vi "scan_save.vi"(6 "Application ref in":refnum<vi>, 7 "Direction: up/down (T=up)":bool, 8 "error in (no error)":errorcluster, 9 "reference 3":refnum<vi>, 10 "reference in":refnum<vi>, 11 "Path in":refnum<vi>) -> ()   [LabVIEW 2019]
uses:
  <userlib>/Nanonis Prog Interface V45/Nanonis Prog Interface.lvlib
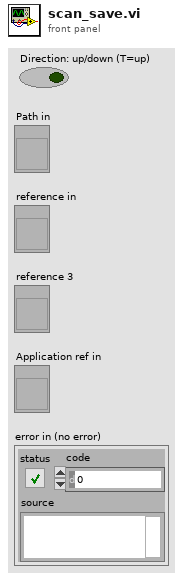
[diagram p1: front panel]
types:
  T1 = cluster{"Scan frame data":sgl[][], "Scan frame data":sgl[][]}
  T2 = cluster{"Scan frame data":sgl[][], "Scan frame data":sgl[][]}[]
  T3 = cluster{"up=T/down=F":bool, "time/line":sgl, "start time":timestamp, "end time":timestamp}
  T4 = cluster{"String":string, "Calibration (per Volt)":sgl, "Offset (physical unit)":sgl, "Channel index":i32}
  T5 = cluster{"Xc":sgl, "Yc":sgl, "Angle (deg)":sgl, "Width":sgl, "Height":sgl, "Pixels/line":i32, "Lines":i32}
  T6 = cluster{"Value":path, "name or relative path":string}
  T7 = cluster{"String":string, "Calibration (per Volt)":sgl, "Offset (physical unit)":sgl, "Channel index":i32}[]
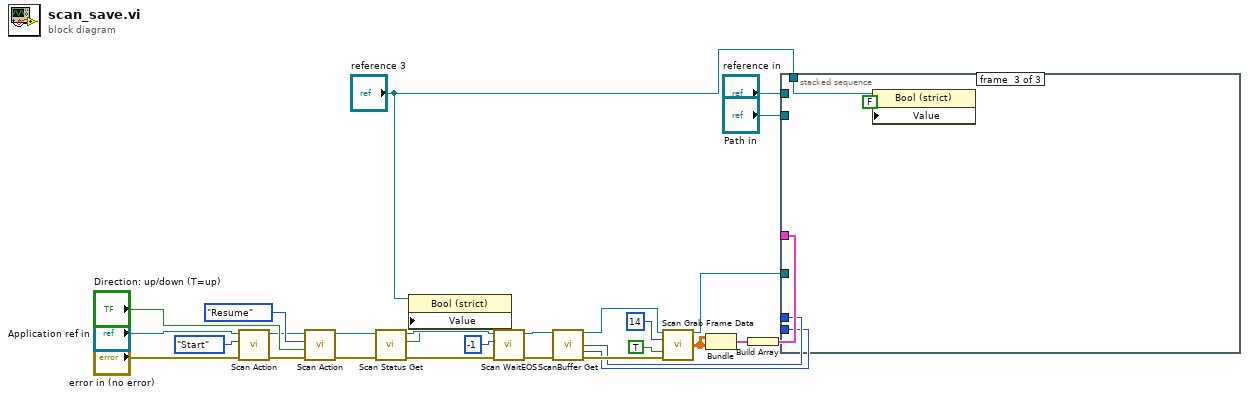
[diagram p0: block diagram]
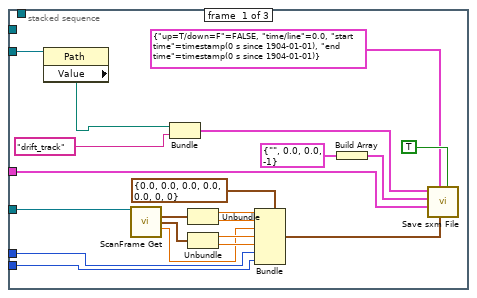
[diagram p2: hidden frame]
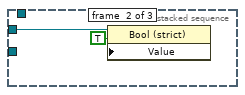
[diagram p3: hidden frame]
diagram:
  n1 = call <userlib>:"Scan Action.vi"("error in (no error)"="error in (no error)", "Scan action (Start)"=enum16{"Start", "Stop", "Pause", "Resume"}."Start", "Application ref in"="Application ref in") -> ("error out"=w11:errorcluster, "Application ref out"=w10:refnum<vi>)  [unwired: 6 in]
  n2 = call <userlib>:"Scan Action.vi"("error in (no error)"=w11, "Direction: up/down (T=up)"="Direction: up/down (T=up)", "Scan action (Start)"=enum16{"Start", "Stop", "Pause", "Resume"}."Resume" ("Scan action"), "Application ref in"=w10) -> ("error out"=w19:errorcluster, "Application ref out"=w20:refnum<vi>)  [unwired: 5 in]
  n3 = call <userlib>:"Scan Status Get.vi"("error in (no error)"=w19, "Application ref in"=w20) -> ("error out"=w7:errorcluster, "Scanning?"=w4:bool, "Application ref out"=w8:refnum<vi>)  [unwired: 6 in]
  n4 = property class="Bool (strict)"(reference="reference 3", "Value"=w4) -> ()  [unwired: 1 in, 2 out]
  n5 = call <userlib>:"Scan WaitEOS.vi"("error in (no error)"=w7, "Timeout in ms (-1)"=-1, "Application ref in"=w8) -> ("error out"=w5:errorcluster, "Application ref out"=w6:refnum<vi>)  [unwired: 4 in, 2 out]
  n6 = call <userlib>:"ScanBuffer Get.vi"("Application ref in"=w6, "error in (no error)"=w5) -> ("Application ref out"=w18:refnum<vi>, "Pixels/line"=w14:i32, "Lines"=w13:i32, "error out"=w17:errorcluster)  [unwired: 9 in, 1 out]
  n7 = call <userlib>:"Scan Grab Frame Data.vi"("Application ref in"=w18, "Channel index (0-23)"=u8 14, "Direction: Fwd/Bwd (T=Fwd)"=TRUE, "error in (no error)"=w17) -> ("Application ref out"=w9:refnum<vi>, "Scan frame data"=w12:sgl[][])  [unwired: 7 in, 3 out]
  n8 = Bundle("Scan frame data"=w12, "Scan frame data"=w12) -> (w16:T1)  [unwired: 1 in]
  n9 = Build Array(w16) -> (w15:T2)
  n10 = stacked-sequence {
    tunnel: w15 -> [w36 _ _]
    tunnel: w9 -> [w35 _ _]
    tunnel: w14 -> [w34 _ _]
    tunnel: w13 -> [w33 _ _]
    tunnel: "Path in" -> [w29 _ _]
    tunnel: "reference in" -> [_ w50 _]
    tunnel: "reference 3" -> [_ _ w52]
    frame #0 {
      n11 = property class="Path"(reference=w29) -> ("Value"=w31:path)  [unwired: 1 in, 2 out]
      n12 = call <userlib>:"ScanFrame Get.vi"("Application ref in"=w35) -> ("Center coordinates (m)"=w37:cluster{"Xc":sgl, "Yc":sgl}, "Size (m)"=w38:cluster{"Width":sgl, "Height":sgl}, "Angle (deg)"=w41:sgl)  [unwired: 10 in, 2 out]
      n13 = Bundle("Value"=w31, "name or relative path"="drift_track") -> (w30:T6)  [unwired: 1 in]
      n14 = Unbundle(w37) -> ("Xc"=w39:sgl, "Yc"=w40:sgl)
      n15 = Unbundle(w38) -> ("Width"=w42:sgl, "Height"=w43:sgl)
      n16 = Bundle(cluster=T5 {"Xc"=0.0, "Yc"=0.0, "Angle (deg)"=0.0, "Width"=0.0, "Height"=0.0, "Pixels/line"=0, "Lines"=0}, "Xc"=w39, "Yc"=w40, "Angle (deg)"=w41, "Width"=w42, "Height"=w43, "Pixels/line"=w34, "Lines"=w33) -> (w45:T5)
      n17 = Build Array(T4 {"String"="", "Calibration (per Volt)"=0.0, "Offset (physical unit)"=0.0, "Channel index"=-1} ("cluster")) -> (w46:T7)
      n18 = call <userlib>:"Save sxm File.vi"("Auto file naming? (T)"=TRUE, "Scanfield"=w45, "Scan param"=T3 {"up=T/down=F"=FALSE, "time/line"=0.0, "start time"=timestamp(0 s since 1904-01-01), "end time"=timestamp(0 s since 1904-01-01)}, "Channels data"=w36, "Channels config"=w46, "Filename control"=w30) -> ()  [unwired: 3 in, 3 out]
    }
    frame #1 {
      n19 = property class="Bool (strict)"(reference=w50, "Value"=TRUE ("Write Result")) -> ()  [unwired: 1 in, 2 out]
    }
    frame #2 {
      n20 = property class="Bool (strict)"(reference=w52, "Value"=FALSE ("Scanning")) -> ()  [unwired: 1 in, 2 out]
    }
  }
